vi "Write TDMS Channel Attributes.vi"(8 "error in (no error)":errorcluster, 10 "TDMS File Ref in":refnum<k34>, 11 "TDMS-Container in":refnum<class "TDMS-Container.lvclass">) -> (0 "error out":errorcluster, 2 "TDMS File Ref out":refnum<k34>, 3 "TDMS-Container out":refnum<class "TDMS-Container.lvclass">)   [LabVIEW 2016, in "BNT_TDMS.lvlib" / "TDMS-Container.lvclass"]
doc: "Write TDMS channel attributes."
uses:
  TDMS-Container.lvclass
  TDMS-Container.lvclass/TDMS-Container.ctl
  TDMSData/TDMS-Data.lvclass
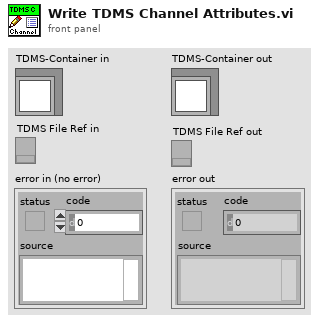
[diagram p1: front panel]
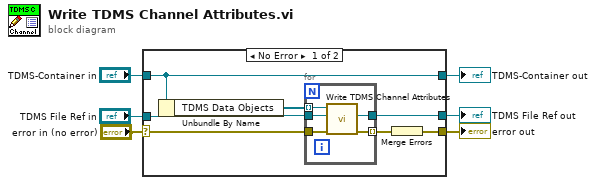
[diagram p0: block diagram]
diagram:
  n1 = case shown="No Error" "error in (no error)" {
    selector: "error in (no error)" -> [w10 w21]
    tunnel: [w7 w21] -> w1
    tunnel: [w13 w20] -> w3
    tunnel: "TDMS-Container in" -> [w13 w20]
    tunnel: "TDMS File Ref in" -> [w11 w19]
    tunnel: [w8 w19] -> w2
    frame No Error {
      n2 = Unbundle By Name(w13) -> ("TDMS Data Objects"=w12:refnum<class "TDMS-Data.lvclass">[])
      n3 = for {
        tunnel: w12 -> [w18] mode=indexing
        tunnel: w11 -> [w16]
        tunnel: w10 -> [w17]
        tunnel: [w14] -> w9 mode=indexing
        tunnel: [w15] -> w8
        n4 = call-dynamic "Write TDMS Channel Attributes.vi"("error in (no error)"=w17, "TDMS File Ref in"=w16, "TDMS-Data in"=w18) -> ("error out"=w14:errorcluster, "TDMS File Ref out"=w15:refnum<k34>)  [unwired: 6 in, 1 out]
      }
      n5 = Merge Errors(w9) -> (w7:errorcluster)
    }
    frame Error {
    }
  }
  "error out" <- w1
  "TDMS-Container out" <- w3
  "TDMS File Ref out" <- w2
